vi "OA_FindAddWorksheet.vi"(5 "Worksheet Name":string, 7 "error in (no error)":errorcluster, 8 "Origin.IOApplication":refnum<k7>) -> (0 "error out":errorcluster, 1 "Found":bool=TRUE, 2 "Origin.Worksheet":refnum<k7>, 3 "Origin.IOApplication":refnum<k7>)   [LabVIEW 2010]
doc: "Find a Worksheet in the current project. If not find, create a new one. \n\nWorksheet Name:\n Name of the Worksheet to find."
panel:
  in  "Origin.Worksheet in":refnum<k7>
  in  "Origin.Worksheet internal":refnum<k7>
  in  "Origin.WorksheetPage Internal":refnum<k7>
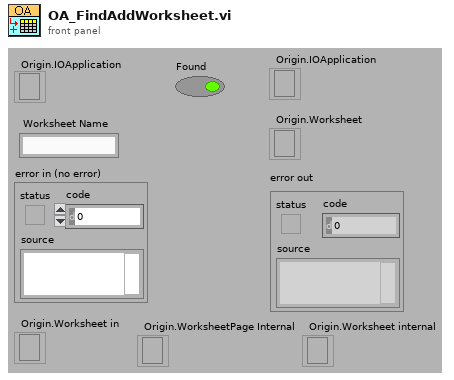
[diagram p1: front panel]
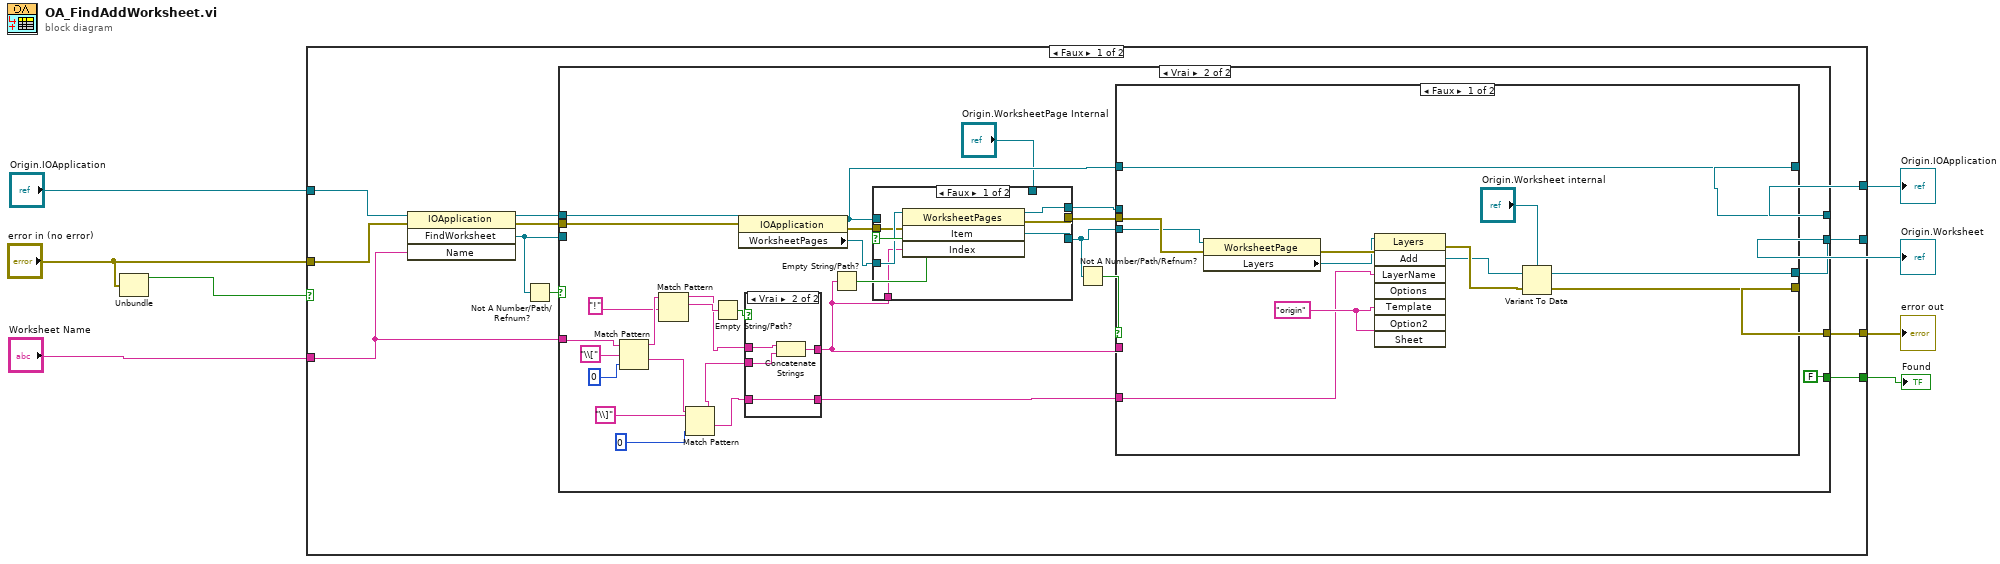
[diagram p0: block diagram]
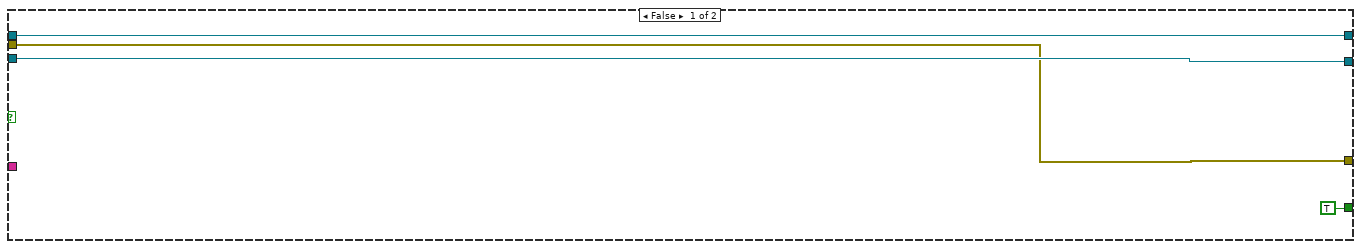
[diagram p2: hidden frame]
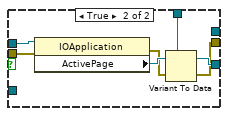
[diagram p3: hidden frame]
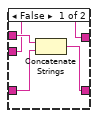
[diagram p4: hidden frame]
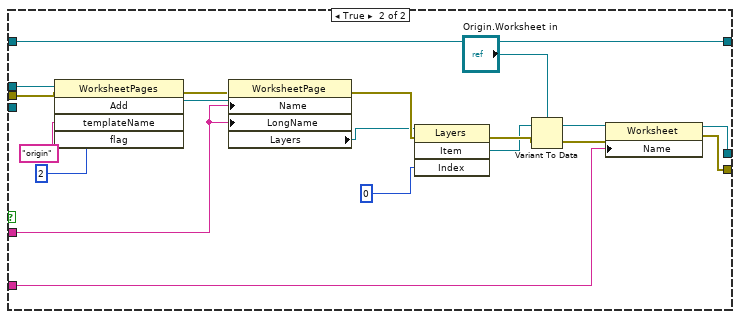
[diagram p5: hidden frame]
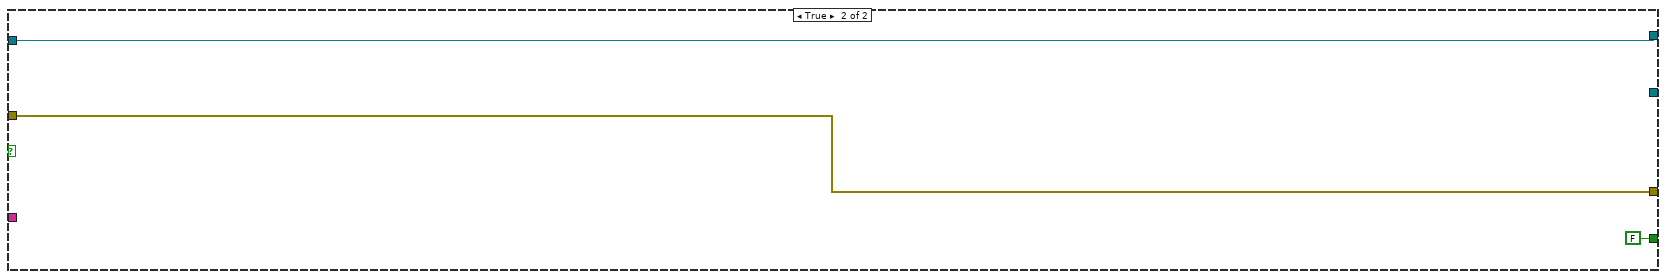
[diagram p6: hidden frame]
diagram:
  n1 = Unbundle("error in (no error)") -> ("status"=w5:bool)  [unwired: 2 out]
  n2 = case shown="Faux" w5 {
    tunnel: "Origin.IOApplication" -> [w19 w108]
    tunnel: "error in (no error)" -> [w18 w107]
    tunnel: "Worksheet Name" -> [w11 _]
    tunnel: [w10 w108] -> w4
    tunnel: [w12 w107] -> w3
    tunnel: [w15 _] -> w2
    tunnel: [w9 FALSE] -> w1
    frame False {
      n3 = invoke class="IOApplication" method="FindWorksheet"(reference=w19, error in=w18, "Name"=w11) -> (reference out=w14:refnum<k7>, error out=w13:errorcluster, "FindWorksheet"=w16:refnum<k7>)  [unwired: 1 in, 1 out]
      n4 = Not A Number/Path/Refnum?(number/path/refnum=w16) -> (NaN/Path/Refnum?=w17:bool)
      n5 = case shown="Vrai" w17 {
        tunnel: w16 -> [w23 _]
        tunnel: [w23 w44] -> w15
        tunnel: w14 -> [w22 w53]
        tunnel: [w22 w42] -> w10
        tunnel: w13 -> [w21 w52]
        tunnel: [w21 w43] -> w12
        tunnel: w11 -> [_ w45]
        tunnel: [TRUE FALSE] -> w9
        frame False {
        }
        frame True {
          n6 = Match Pattern(string=w45, regular expression="\\[", offset (0)=0) -> (before substring=w41:string, after substring=w48:string)  [unwired: 2 out]
          n7 = Match Pattern(string=w41, regular expression="!") -> (before substring=w37:string, match substring=w38:string)  [unwired: 1 in, 2 out]
          n8 = Match Pattern(string=w48, regular expression="\\]", offset (0)=0) -> (before substring=w36:string, after substring=w35:string)  [unwired: 2 out]
          n9 = Empty String/Path?(string/path=w38) -> (empty?=w39:bool)
          n10 = property class="IOApplication"(reference=w53, error in=w52) -> (reference out=w32:refnum<k7>, error out=w31:errorcluster, "WorksheetPages"=w29:refnum<k7>)
          n11 = case shown="Vrai" w39 {
            tunnel: w36 -> [w67 w73]
            tunnel: w37 -> [w70 w74]
            tunnel: [w67 w72] -> w26
            tunnel: w35 -> [w69 w71]
            tunnel: [w68 w71] -> w34
            frame False {
              n12 = Concatenate Strings(w70, w69) -> (w68:string)
            }
            frame True {
              n13 = Concatenate Strings(w74, w73) -> (w72:string)
            }
          }
          n14 = Empty String/Path?(string/path=w26) -> (empty?=w33:bool)
          n15 = case shown="Faux" w33 {
            tunnel: w32 -> [_ w66]
            tunnel: w31 -> [w58 w65]
            tunnel: [w56 w60] -> w30
            tunnel: [w55 w61] -> w27
            tunnel: w29 -> [w59 _]
            tunnel: w26 -> [w57 _]
            tunnel: "Origin.WorksheetPage Internal" -> [_ w62]
            tunnel: [w54 _] -> w25
            frame False {
              n16 = invoke class="WorksheetPages" method="Item"(reference=w59, error in=w58, "Index"=w57) -> (reference out=w54:refnum<k7>, error out=w56:errorcluster, "Item"=w55:refnum<k7>)  [unwired: 1 in, 1 out]
            }
            frame True {
              n17 = property class="IOApplication"(reference=w66, error in=w65) -> (error out=w63:errorcluster, "ActivePage"=w64:refnum<k7>)  [unwired: 1 out]
              n18 = Variant To Data(error in=w63, Variant=w64, type=w62) -> (error out=w60:errorcluster, data=w61:refnum<k7>)
            }
          }
          n19 = Not A Number/Path/Refnum?(number/path/refnum=w27) -> (NaN/Path/Refnum?=w51:bool)
          n20 = case shown="Faux" w51 {
            tunnel: w34 -> [w81 w90]
            tunnel: w30 -> [w80 w94]
            tunnel: w27 -> [w79 _]
            tunnel: [w77 w88] -> w44
            tunnel: [w76 w89] -> w43
            tunnel: w32 -> [w75 w87]
            tunnel: [w75 w87] -> w42
            tunnel: w25 -> [_ w93]
            tunnel: w26 -> [_ w92]
            frame False {
              w85 = "origin"
              n21 = property class="WorksheetPage"(reference=w79, error in=w80) -> (error out=w86:errorcluster, "Layers"=w78:refnum<k7>)  [unwired: 1 out]
              n22 = invoke class="Layers" method="Add"(reference=w78, error in=w86, "LayerName"=w81, "Template"=w85, "Sheet"=w85) -> (error out=w84:errorcluster, "Add"=w83:refnum<k7>)  [unwired: 3 in, 6 out]
              n23 = Variant To Data(error in=w84, Variant=w83, type="Origin.Worksheet internal") -> (error out=w76:errorcluster, data=w77:refnum<k7>)
            }
            frame True {
              n24 = invoke class="WorksheetPages" method="Add"(reference=w93, error in=w94, "templateName"="origin", "flag"=2) -> (error out=w104:errorcluster, "Add"=w105:refnum<k7>)  [unwired: 1 in, 3 out]
              n25 = property class="WorksheetPage"(reference=w105, error in=w104, "Name"=w92, "LongName"=w92) -> (error out=w101:errorcluster, "Layers"=w99:refnum<k7>)  [unwired: 1 out]
              n26 = invoke class="Layers" method="Item"(reference=w99, error in=w101, "Index"=0) -> (error out=w98:errorcluster, "Item"=w97:refnum<k7>)  [unwired: 1 in, 2 out]
              n27 = Variant To Data(error in=w98, Variant=w97, type="Origin.Worksheet in") -> (error out=w91:errorcluster, data=w95:refnum<k7>)
              n28 = property class="Worksheet"(reference=w95, error in=w91, "Name"=w90) -> (reference out=w88:refnum<k7>, error out=w89:errorcluster)
            }
          }
        }
      }
    }
    frame True {
    }
  }
  "Origin.IOApplication" <- w4
  "error out" <- w3
  "Origin.Worksheet" <- w2
  "Found" <- w1
